vi "FGV_Stop.vi"(7 "Get/Set":T1, 11 "STOP in":bool) -> (3 "STOP out":bool)   [LabVIEW 2019]
uses:
  TypeDef/#TypeDef_SetGet.ctl
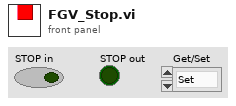
[diagram p1: front panel]
types:
  T1 = typedef "#TypeDef_SetGet.ctl" = enum16{"Set", "Get"}
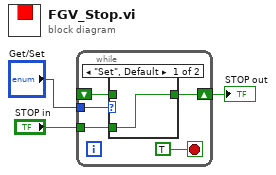
[diagram p0: block diagram]
diagram:
  n1 = while {
    tunnel: "Get/Set" -> [w7]
    shift-right: [w4] -> w3
    shift-left: _ -> [w6]
    tunnel: "STOP in" -> [w5]
    stop <- TRUE stop-if-true
    n2 = case shown="\"Set\", Default" w7 {
      tunnel: w6 -> [_ w10]
      tunnel: w5 -> [w9 _]
      tunnel: [w9 w10] -> w4
      frame "Set", Default {
      }
      frame "Get" {
      }
    }
  }
  "STOP out" <- w3
